vi "dfd_FXP PtByPt AntiSymmetric FIR.vi"(6 "state in":i64[](array[numeric]), 7 "FXPOPs":T5[](array[typedef]) {"source" items=["Coef a/k"=0, "Coef b/v"=7, "Input"=1, "Output"=2, "Multiplicand"=3, "Product"=4, "Sum"=5, "Delay"=6, "Gain"=8]}, 8 "filtering statistics in":T3(array[cluster]) {"statistics information"."min value" format="%.2f"; "statistics information"."max value" format="%.2f"; "Quantizer Source" items=["Coefficients a/k"=0, "Coefficients b/v"=7, "Input"=1, "Output"=2, "Multiplicand"=3, "Product"=4, "Sum"=5, "Delay"=6]}, 10 "coef b (half storage)":T4, 11 "x":T7={"value"=0, "wl"=0, "iwl"=0, "Signed"=TRUE} {"value" format="%.0x"}) -> (0 "filtering statistics out":T3(array[cluster]) {"statistics information"."min value" format="%.2f"; "statistics information"."max value" format="%.2f"; "Quantizer Source" items=["Coefficients a/k"=0, "Coefficients b/v"=7, "Input"=1, "Output"=2, "Multiplicand"=3, "Product"=4, "Sum"=5, "Delay"=6]}, 3 "filtered x":T7={"value"=0, "wl"=0, "iwl"=0, "Signed"=TRUE} {"value" format="%.0x"}, 4 "state out":i64[](array[numeric]))   [LabVIEW 2017, in "NI_DigFilter_FXP.lvlib"]
uses:
  <vilib>/addons/Digital Filter Design/NI_DigFilter_FXP.lvlib
  <vilib>/addons/Digital Filter Design/_Objects.llb/dfd_DFXP Data Type (scaler).ctl
  <vilib>/addons/Digital Filter Design/_Objects.llb/dfd_DFXP Operation Parameter.ctl
  <vilib>/addons/Digital Filter Design/_Objects.llb/dfd_Internal Quantization Srcs.ctl
  <vilib>/addons/Digital Filter Design/_Objects.llb/dfd_DFXP Data Type (vector).ctl
  <vilib>/addons/Digital Filter Design/_Objects.llb/DFD Quantization Sources.ctl
  <vilib>/addons/Digital Filter Design/_Objects.llb/DFD FXP Statistics Data.ctl
  <vilib>/addons/Digital Filter Design/NI_DigFilterLicensed.lvlib
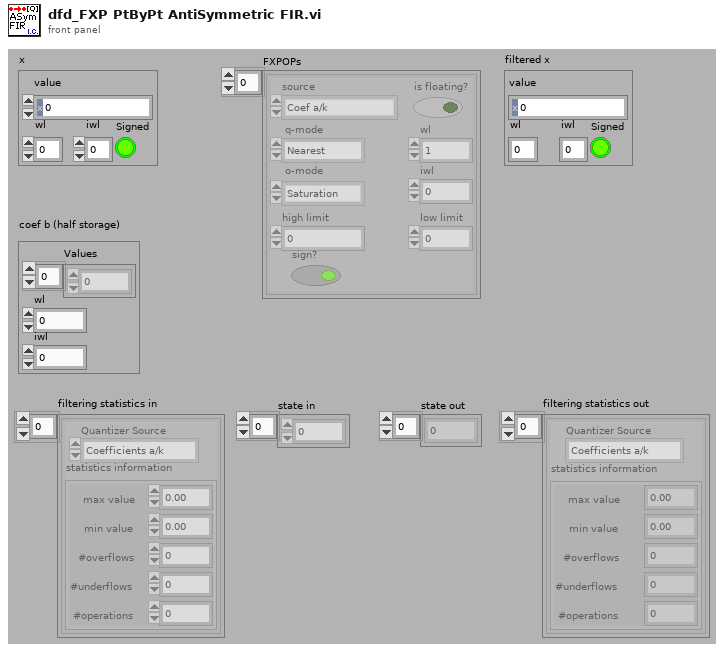
[diagram p1: front panel]
types:
  T1 = typedef "NI_DigFilterLicensed.lvlib/DFD Quantization Sources.ctl" = u16
  T2 = typedef "NI_DigFilterLicensed.lvlib/DFD FXP Statistics Data.ctl" = cluster{"max value":ext, "min value":ext, "#overflows":i32, "#underflows":i32, "#operations":i32}
  T3 = cluster{"Quantizer Source":T1, "statistics information":T2}[]
  T4 = typedef "dfd_DFXP Data Type (vector).ctl" = cluster{"Values":i64[], "wl":i16, "iwl":i16}
  T5 = typedef "dfd_DFXP Operation Parameter.ctl" = cluster{"source":T6, "is floating?":bool, "o-mode":enum16{"Saturation", "Wrap"}, "q-mode":enum16{"Nearest", "Truncation"}, "wl":i16, "high limit":i64, "low limit":i64, "iwl":i16, "sign?":bool}
  T6 = typedef "NI_DigFilterLicensed.lvlib/dfd_Internal Quantization Srcs.ctl" = u16
  T7 = typedef "dfd_DFXP Data Type (scaler).ctl" = cluster{"value":i64, "wl":i16, "iwl":i16, "Signed":bool}
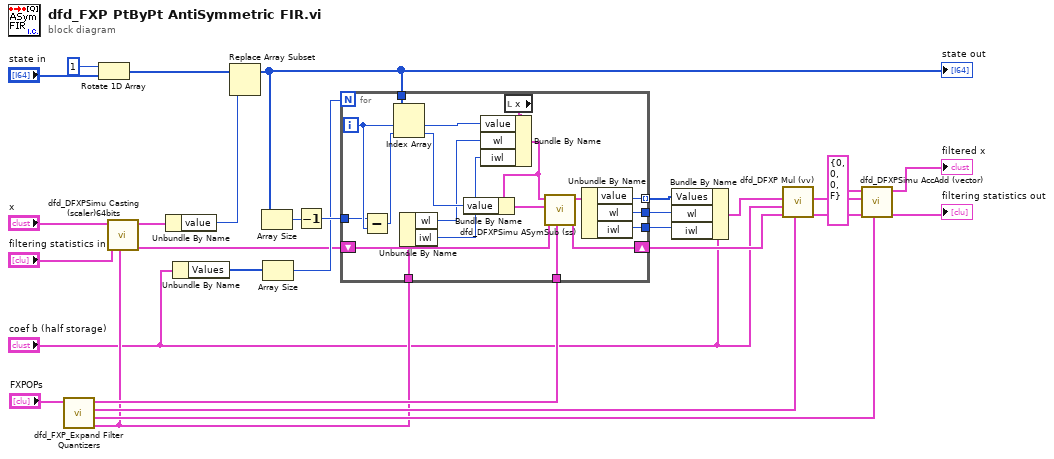
[diagram p0: block diagram]
diagram:
  n1 = call <vilib>:"dfd_FXP_Expand Filter Quantizers.vi"("FXPOPs"="FXPOPs") -> ("Delay"=w5:T5, "Sum"=w15:T5, "Product"=w16:T5, "Multiplicand"=w12:T5)  [unwired: 7 out]
  n2 = Rotate 1D Array(1:"state in", 2:1 ("n")) -> (0:w28:i64[])
  n3 = call <vilib>:"dfd_DFXPSimu Casting (scaler)64bits.vi"("op params"=w5, "filtering statistics in"="filtering statistics in", "Value in"="x") -> ("filtering statistics out"=w11:T3, "Value out"=w26:T7)  [unwired: 1 in, 6 out]
  n4 = Unbundle By Name(w26) -> ("value"=w7:i64)
  n5 = Unbundle By Name("coef b (half storage)") -> ("Values"=w6:i64[])
  n6 = Replace Array Subset(array=w28, new element=w7) -> (w25:i64[])  [unwired: 1 in]
  "state out" <- w25
  n7 = Array Size(array=w25) -> (size(s)=w24:i32)
  n8 = Array Size(array=w6) -> (size(s)=w13:i32)
  n9 = Decrement(x=w24) -> (x-1=w22:i32)
  n10 = for {
    N: w13 -> [_]
    tunnel: w25 -> [w48]
    tunnel: w22 -> [w45]
    tunnel: [w32] -> w9 mode=indexing
    tunnel: w12 -> [w41]
    shift-right: [w39] -> w10
    shift-left: w11 -> [w40]
    tunnel: w5 -> [w37]
    tunnel: [w31] -> w2
    tunnel: [w30] -> w1
    i -> [w47]
    n11 = Subtract(x=w45, y=w47) -> (x-y=w46:i32)
    n12 = Index Array(array=w48, index #1=w47, index #2=w46) -> (element #1=w43:i64, element #2=w42:i64)
    n13 = Unbundle By Name(w37) -> ("wl"=w36:i16, "iwl"=w35:i16)
    n14 = local read "x"() -> (w38:T7)
    n15 = Bundle By Name(cluster=w38, "value"=w43, "wl"=w36, "iwl"=w35) -> (w33:T7)
    n16 = Bundle By Name(cluster=w33, "value"=w42) -> (w34:T7)
    n17 = call <vilib>:"dfd_DFXPSimu ASymSub (ss).vi"("op params"=w41, "filtering statistics in"=w40, "value2 in"=w34, "value1 in"=w33) -> ("filtering statistics out"=w39:T3, "value out"=w44:T7)  [unwired: 1 in, 5 out]
    n18 = Unbundle By Name(w44) -> ("value"=w32:i64, "wl"=w31:i16, "iwl"=w30:i16)
  }
  n19 = Bundle By Name(cluster="coef b (half storage)", "Values"=w9, "wl"=w2, "iwl"=w1) -> (w4:T4)
  n20 = call <vilib>:"dfd_DFXP Mul (vv).vi"("op params"=w16, "filtering statistics in"=w10, "Value in 2"="coef b (half storage)", "Value in"=w4) -> ("filtering statistics out"=w21:T3, "Value out"=w19:T4)  [unwired: 6 out]
  n21 = call <vilib>:"dfd_DFXPSimu AccAdd (vector).vi"("op params"=w15, "filtering statistics in"=w21, "addends"=w19, "acc in"=T7 {"value"=0, "wl"=0, "iwl"=0, "Signed"=FALSE}) -> ("filtering statistics out"=→"filtering statistics out":T3, "acc out"=→"filtered x":T7)  [unwired: 1 in, 5 out]
